vi "PS_Signal_Gen_Write.vi"(10 "Value String":string, 11 "Command String":string) -> (0 "error out":errorcluster)   [LabVIEW 2011]
uses:
  PS_Global.vi
  <vilib>/Instr/_visa.llb/VISA Configure Serial Port (Instr).vi
panel:
  in  "baud rate":u32=115200
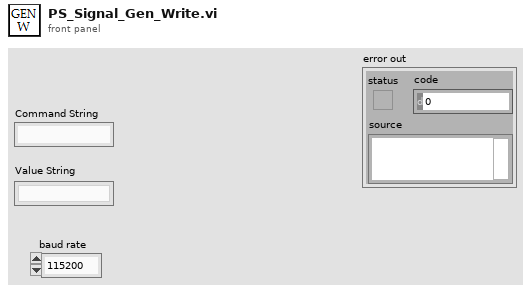
[diagram p1: front panel]
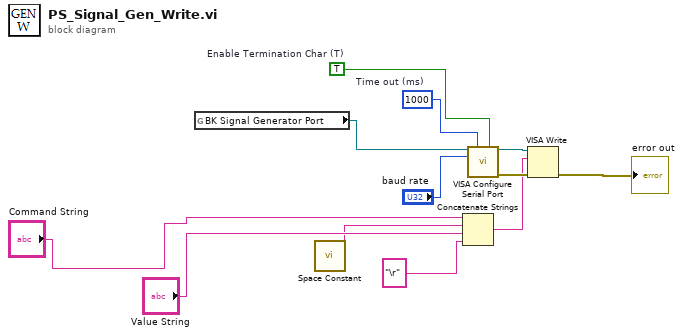
[diagram p0: block diagram]
diagram:
  w8 = TRUE  # Enable Termination Char (T)
  w11 = 1000  # Time out (ms)
  n1 = global read "PS_Global.vi" "BK Signal Generator Port"() -> (w6:refnum<visa-resource-name>)
  n2 = call <vilib>:"Space Constant.vi"() -> ("String"=w2:string)
  n3 = Concatenate Strings("Command String", w2, "Value String", "\r") -> (w7:string)
  n4 = call-poly "VISA Configure Serial Port"("VISA resource name"=w6, "timeout (10sec)"=w11, "Enable Termination\nChar (T)"=w8, "baud rate (9600)"="baud rate") -> ("VISA resource name out"=w10:refnum<visa-resource-name>, "error out"=w9:errorcluster)  [unwired: 10 in]
  n5 = VISA Write(VISA resource name=w10, write buffer=w7, error in (no error)=w9) -> (error out=→"error out":errorcluster)  [unwired: 2 out]
